vi "conti_move_v2.0.vi"(7 "enable":bool, 8 "error in (no error)":errorcluster, 9 "Position":T1, 11 "route":T2[](array[typedef])) -> (0 "error out":errorcluster, 1 "Position out":T1)   [LabVIEW 2019]
uses:
  move_cluster.ctl
  move/position cluster.ctl
  <vilib>/Platform/TimedLoop/XDataNode/timing_clust.ctl
  <vilib>/Platform/TimedLoop/XDataNode/nitl_modes.ctl
  <vilib>/Platform/TimedLoop/XDataNode/wakeup.ctl
  <vilib>/platform/TimedLoop/XDataNode/XDataNode.xnode
  <vilib>/Platform/TimedLoop/XDataNode/XDNodeRunTimeDep.lvlib
panel:
  out "Waveform Chart":cluster{"yaw":dbl, dbl}(graph)
  out "x-y":u32
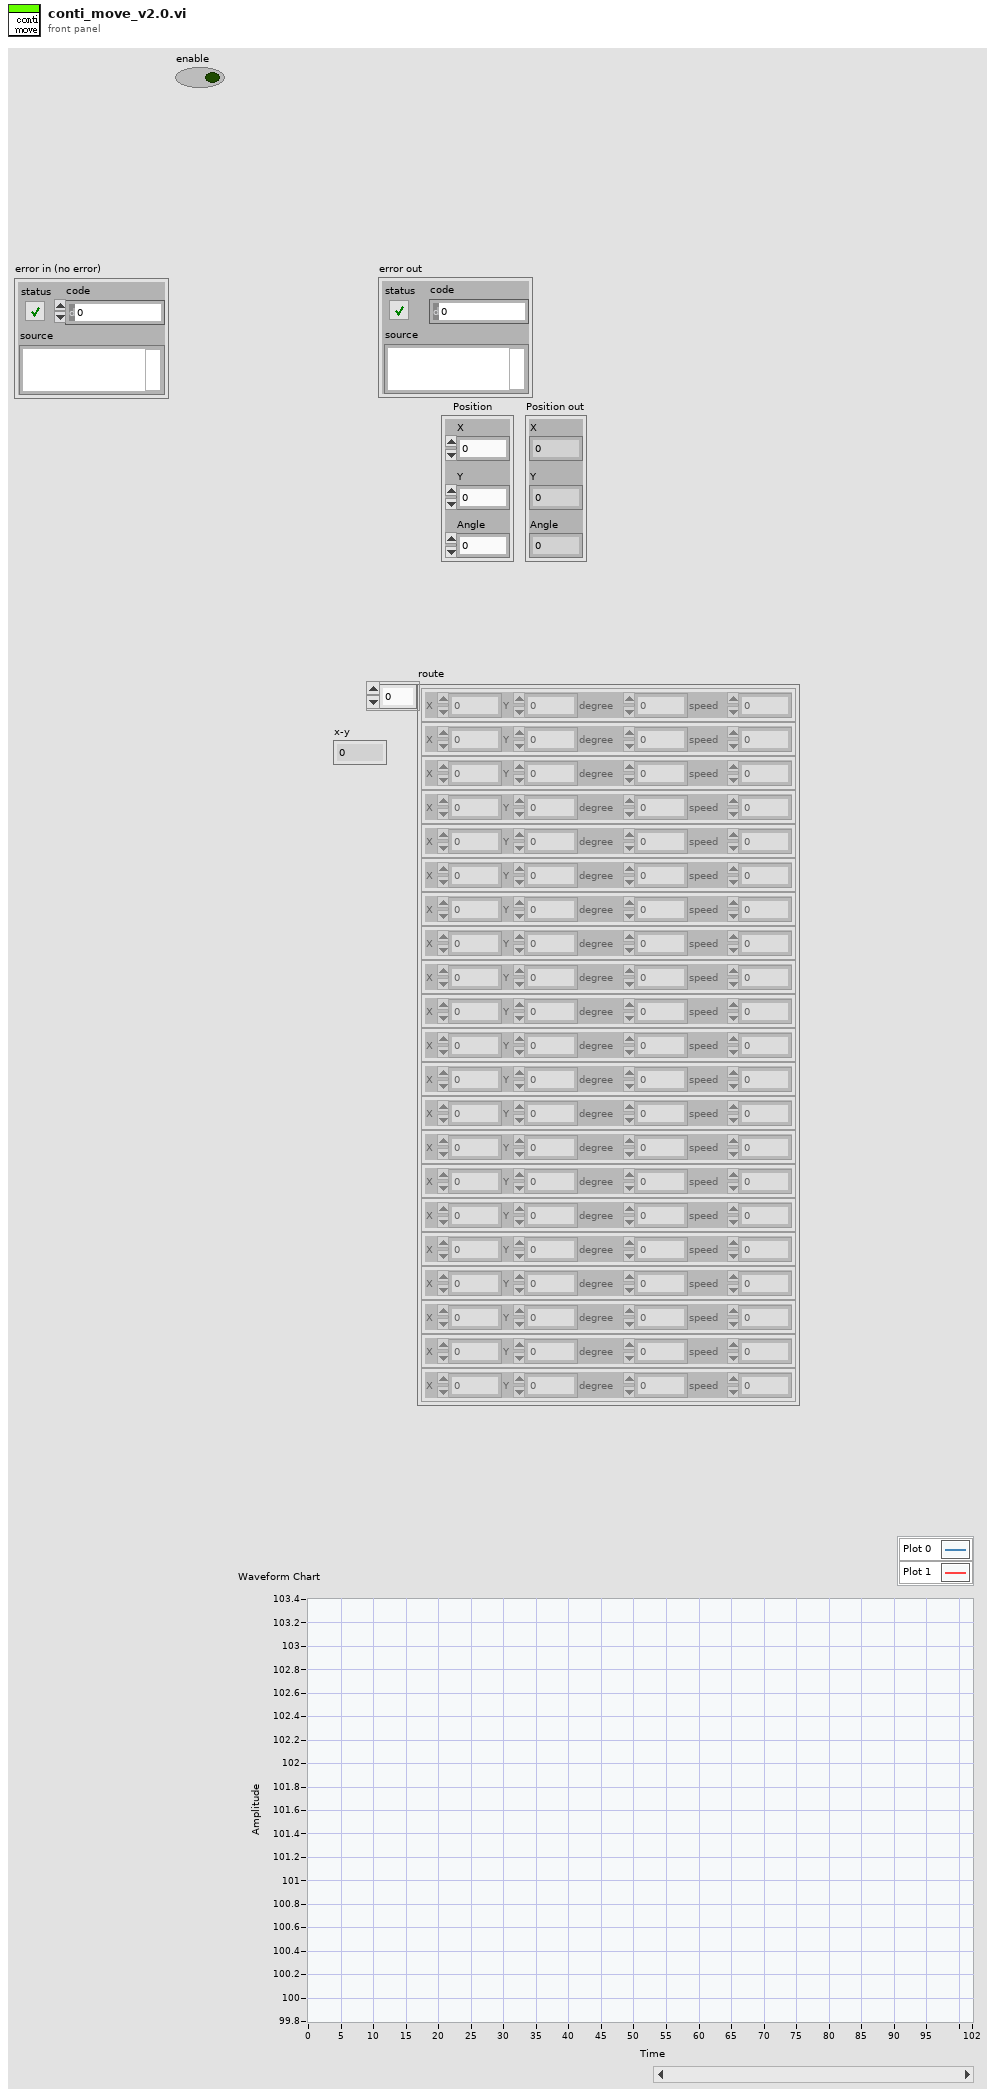
[diagram p1: front panel]
types:
  T1 = typedef "position cluster.ctl" = cluster{"X":dbl, "Y":dbl, "Angle":dbl}
  T2 = typedef "move_cluster.ctl" = cluster{"X":dbl, "Y":dbl, "degree":dbl, "speed":dbl}
  T3 = typedef "BNO055 gyro 3axis.ctl" = cluster{"yaw":dbl, "pitch":dbl, "roll":dbl}
  T4 = typedef "XDNodeRunTimeDep.lvlib/timing_clust.ctl" = cluster{"Expected End [f-1]":u64, "Actual End [f-1]":u64, "Finished Late? [f-1]":bool, "Expected End [i-1]":u64, "Actual End [i-1]":u64, "Finished Late? [i-1]":bool, "Expected Start [i]":u64, "Actual Start [i]":u64, "Expected Start [f]":u64, "Actual Start [f]":u64, "Source Name":string, "Structure Name":string, "Period":i64, "Deadline":i64, "Offset":i64, "Start":i64, "Priority":i32, "Timeout":i32, "Mode":T5, "Wakeup Reason":T6, "Error":errorcluster, "Source Type":string, "Secondary Source Type":string, "Global End Time":u64, "Global Start Time":u64, "Frame Duration":u64, "Iteration Duration":u64, "Assigned CPU":i32, "I/O Scan Engine Mode":u32}
  T5 = typedef "XDNodeRunTimeDep.lvlib/nitl_modes.ctl" = enum32{"No Change", "Process missed periods, maintain original phase", "Discard missed periods, maintain original phase", "Process missed periods, ignore original phase", "Discard missed periods, ignore original phase"}
  T6 = typedef "XDNodeRunTimeDep.lvlib/wakeup.ctl" = enum32{"Normal", "Aborted", "Asynchronous wakeup", "Timing source error", "Timed loop error", "Timeout"}
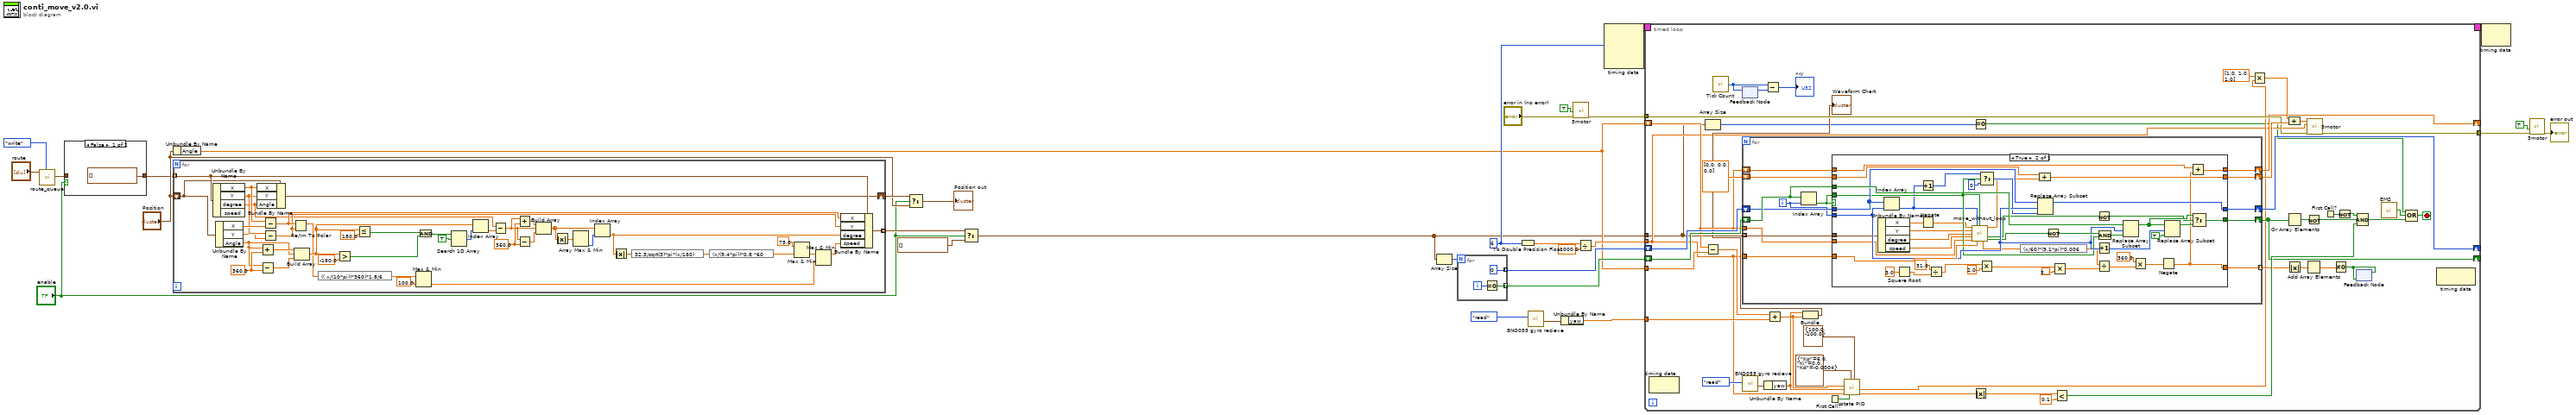
[diagram p0: block diagram]
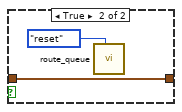
[diagram p2: hidden frame]
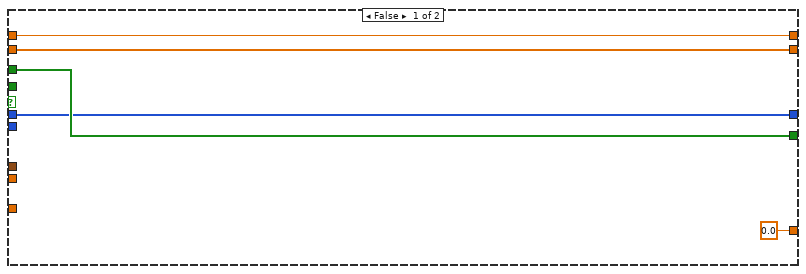
[diagram p3: hidden frame]
diagram:
  w27 = i64 6 ("Period")
  n1 = call "route_queue.vi"("set"=enum16{"reset", "write"}."write", "route"="route") -> ("read"=w2:T2[])  [unwired: 9 in]
  n2 = case shown="False" "enable" {
    tunnel: w2 -> [_ w33]
    tunnel: [T2[] [] ("read") w33] -> w3
    frame False {
    }
    frame True {
      n3 = call "route_queue.vi"("set"=enum16{"reset", "write"}."reset") -> ()  [unwired: 10 in, 1 out]
    }
  }
  n4 = Unbundle By Name("Position") -> ("Angle"=w12:dbl)
  n5 = for {
    tunnel: w3 -> [w75] mode=indexing
    tunnel: [w74] -> w9 mode=indexing
    shift-right: [w39] -> w10
    shift-left: "Position" -> [w73]
    w61 = 360.0
    w72 = 360.0
    n6 = Unbundle By Name(w75) -> ("X"=w53:dbl, "Y"=w51:dbl, "degree"=w38:dbl)  [unwired: 1 out]
    n7 = Unbundle By Name(w73) -> ("X"=w52:dbl, "Y"=w50:dbl, "Angle"=w54:dbl)
    n8 = Bundle By Name(cluster=w73, "X"=w53, "Y"=w51, "Angle"=w38) -> (w39:T1)
    n9 = Add(x=w54, y=w72) -> (x+y=w71:dbl)
    n10 = Subtract(x=w54, y=w72) -> (x-y=w70:dbl)
    n11 = Subtract(x=w53, y=w52) -> (x-y=w46:dbl)
    n12 = Subtract(x=w51, y=w50) -> (x-y=w45:dbl)
    n13 = Re/Im To Polar(2:w45, 3:w46) -> (1:w44:dbl)  [unwired: 1 out]
    n14 = Build Array(w71, w54, w70) -> (w62:dbl[])
    n15 = expression code="(( x/(10*pi))*360)*1.8/6"(w44) -> (w41:dbl)
    n16 = Greater?(x=w62, y=-180.0) -> (0:w66:bool[])
    n17 = Less Or Equal?(x=w62, y=180.0) -> (x <= y?=w67:bool[])
    n18 = Max & Min(x=w41, y=100.0) -> (min(x,y)=w36:dbl)  [unwired: 1 out]
    n19 = And(x=w67, y=w66) -> (x .and. y?=w65:bool[])
    n20 = Search 1D Array(1D array=w65, element=TRUE) -> (index of element=w63:i32)  [unwired: 1 in]
    n21 = Index Array(array=w62, index=w63) -> (element=w37:dbl)
    n22 = Subtract(x=w38, y=w37) -> (x-y=w59:dbl)
    n23 = Add(x=w59, y=w61) -> (x+y=w60:dbl)
    n24 = Subtract(x=w59, y=w61) -> (x-y=w58:dbl)
    n25 = Build Array(w60, w59, w58) -> (w55:dbl[])
    n26 = Absolute Value(x=w55) -> (abs(x)=w57:dbl[])
    n27 = Array Max & Min(array=w57) -> (min index (indices)=w56:i32)  [unwired: 3 out]
    n28 = Index Array(array=w55, index=w56) -> (element=w47:dbl)
    n29 = Absolute Value(x=w47) -> (abs(x)=w48:dbl)
    n30 = expression code="32.3/sqrt(3)*pi*(x/180)"(w48) -> (w49:dbl)
    n31 = expression code="(x/(9.4*pi))*0.8 *60"(w49) -> (w43:dbl)
    n32 = Max & Min(x=75.0, y=w43) -> (min(x,y)=w35:dbl)  [unwired: 1 out]
    n33 = Max & Min(x=w35, y=w36) -> (max(x,y)=w34:dbl)  [unwired: 1 out]
    n34 = Bundle By Name(cluster=w75, "X"=w46, "Y"=w45, "degree"=w47, "speed"=w34) -> (w74:T2)
  }
  n35 = Select(t=w10, s="enable", f="Position") -> (s? t:f=→"Position out":T1)
  n36 = Select(t=w9, s="enable", f=T2[] []) -> (s? t:f=w1:T2[])
  n37 = Array Size(array=w1) -> (size(s)=w23:i32)
  n38 = for {
    N: w23 -> [_]
    tunnel: [w76] -> w24 mode=indexing
    tunnel: [0 ("Boolean")] -> w22 mode=indexing
    i -> [w77]
    n39 = Equal To 0?(x=w77) -> (x = 0?=w76:bool)
  }
  n40 = To Double Precision Float(number=w27) -> (double precision float=w28:dbl)
  n41 = call "BNO055 gyro recieve.vi"("Enum"=enum16{"read", "write"}."read") -> ("read"=w14:T3)  [unwired: 10 in]
  n42 = Unbundle By Name(w14) -> ("yaw"=w13:dbl)
  n43 = call "3motor.vi"("error in (no error)"="error in (no error)", "Reset"=TRUE) -> ("error out"=w19:errorcluster)  [unwired: 8 in, 1 out]
  n44 = Divide(x=w28, y=1000.0) -> (x/y=w25:dbl)
  n45 = node-c288(w27) -> (w30:T4)  [unwired: 3 in]
  n46 = timed-loop {
    timing: w30 -> [_]
    timing-out: [_] -> w29
    tunnel: w25 -> [w82]
    shift-right: [w103] -> _
    shift-left: w24 -> [w125]
    shift-right: [w123] -> _
    shift-left: w22 -> [w124]
    shift-right: [w96] -> _
    shift-left: w12 -> [w111]
    tunnel: w1 -> [w81]
    tunnel: [w121] -> w21
    tunnel: w19 -> [w112]
    tunnel: w13 -> [w92]
    tunnel: w12 -> [w88]
    stop <- w117 stop-if-true
    n47 = node-c288() -> ()  [unwired: 1 in, 1 out]
    n48 = Array Size(array=w81) -> (size(s)=w80:i32)
    n49 = Subtract(x=w111, y=w88) -> (x-y=w89:dbl)
    n50 = call "Tick Count"() -> ("Tick Count(uSec)"=w106:u32)
    n51 = feedback-in #1(w106) -> ()
    n52 = feedback #1() -> (w105:u32)  [unwired: 1 in]
    n53 = for {
      tunnel: w82 -> [w139]
      shift-right: [w136] -> w103
      shift-left: w125 -> [w138]
      shift-right: [w132] -> w123
      shift-left: w124 -> [w137]
      shift-right: [w134] -> w120
      shift-left: dbl[] [0.0, 0.0, 0.0] -> [w133]
      shift-right: [w131] -> w96
      shift-left: w111 -> [w129]
      tunnel: w81 -> [w130] mode=indexing
      tunnel: [w128] -> w100 mode=indexing
      tunnel: w111 -> [w127]
      i -> [w135]
      n54 = Index Array(array=w138, index=w135) -> (element=w126:bool)
      n55 = case shown="True" w126 {
        tunnel: w139 -> [_ w190]
        tunnel: w138 -> [w144 w189]
        tunnel: w137 -> [w143 w188]
        tunnel: [w144 w186] -> w136
        tunnel: w135 -> [_ w181]
        tunnel: [w142 w178] -> w134
        tunnel: w133 -> [w142 w177]
        tunnel: w126 -> [_ w175]
        tunnel: [w143 w172] -> w132
        tunnel: [w141 w164] -> w131
        tunnel: w130 -> [_ w162]
        tunnel: w129 -> [w141 w149]
        tunnel: [0.0 w148] -> w128
        tunnel: w127 -> [_ w145]
        frame False {
        }
        frame True {
          n56 = Unbundle By Name(w162) -> ("X"=w147:dbl, "Y"=w160:dbl, "degree"=w159:dbl, "speed"=w161:dbl)
          n57 = Index Array(array=w188, index=w181) -> (element=w173:i32)
          n58 = Square Root(x=3.0) -> (sqrt(x)=w170:dbl)
          n59 = Increment(x=w173) -> (x+1=w174:i32)
          n60 = Negate(x=w147) -> (-x=w146:dbl)
          n61 = Divide(x=31.0, y=w170) -> (x/y=w168:dbl)
          n62 = call "move_without_loop.vi"("X"=w146, "i"=w173, "run"=w175, "Y"=w160, "deg"=w159, "speed"=w161, "offset"=w145, "dt"=w190) -> ("speed out"=w156:dbl[], "t2?"=w179:bool, "rotate speed"=w154:dbl, "complet"=w157:bool)  [unwired: 3 in, 1 out]
          n63 = Multiply(x=w168, y=2.0) -> (x*y=w165:dbl)
          n64 = Select(t=w174, s=w175, f=0) -> (s? t:f=w176:i32)
          n65 = expression code="(x/60)*(9.1*pi)*0.006"(w154) -> (w152:dbl)
          n66 = Replace Array Subset(array=w188, new element=w176, index=w181) -> (w172:i32[])
          n67 = Compound Arithmetic op=ADD(w177, w156) -> (w178:dbl[])
          n68 = Not(x=w157) -> (.not. x?=w187:bool)
          n69 = Multiply(x=w165, y=3.141592653589793) -> (x*y=w153:dbl)
          n70 = Not(x=w179) -> (.not. x?=w183:bool)
          n71 = Increment(x=w181) -> (x+1=w182:i32)
          n72 = Divide(x=w152, y=w153) -> (x/y=w163:dbl)
          n73 = Compound Arithmetic op=AND(w187, w175) -> (w158:bool)
          n74 = Replace Array Subset(array=w189, new element=w158, index=w181) -> (w185:bool[])
          n75 = Multiply(x=360.0, y=w163) -> (x*y=w151:dbl)
          n76 = Negate(x=w151) -> (-x=w148:dbl)
          n77 = Replace Array Subset(array=w185, new element=TRUE, index=w182) -> (w184:bool[])
          n78 = Add(x=w149, y=w148) -> (x+y=w164:dbl)
          n79 = Select(t=w185, s=w183, f=w184) -> (s? t:f=w186:bool[])
        }
      }
    }
    n80 = call "BNO055 gyro recieve.vi"("Enum"=enum16{"read", "write"}."read") -> ("read"=w91:T3)  [unwired: 10 in]
    n81 = Unbundle By Name(w91) -> ("yaw"=w85:dbl)
    n82 = Subtract(x=w106, y=w105) -> (x-y=→"x-y":u32)
    n83 = Add(x=w89, y=w92) -> (x+y=w84:dbl)
    n84 = Bundle("yaw"=w85, w84) -> (→"Waveform Chart":cluster{"yaw":dbl, dbl})  [unwired: 1 in]
    n85 = First Call?() -> (First Call?: T/F=w93:bool)
    n86 = call "rotate PID.vi"("output range"=cluster{"output high":dbl, "output low":dbl} {"output high"=100.0, "output low"=-100.0}, "s"=w93, "PID"=cluster{"Kp":dbl, "Ki":dbl, "Kd":dbl} {"Kp"=6.0, "Ki"=0.0, "Kd"=-0.0004}, "dt (s)"=w82, "Processer"=w85, "setpoint"=w84) -> ("e(t)"=w83:dbl, "out"=w87:dbl)  [unwired: 4 in]
    n87 = Equal To 0?(x=w80) -> (x = 0?=w79:bool)
    n88 = Absolute Value(x=w83) -> (abs(x)=w110:dbl)
    n89 = Less?(x=w110, y=0.1) -> (x < y?=w108:bool)
    n90 = Multiply(x=dbl[] [1.0, 1.0, 1.0], y=w87) -> (x*y=w118:dbl[])
    n91 = Or Array Elements(Boolean array=w103) -> (logical OR=w102:bool)
    n92 = Absolute Value(x=w100) -> (abs(x)=w99:dbl[])
    n93 = Compound Arithmetic op=ADD(w118, w120) -> (w107:dbl[])
    n94 = Add Array Elements(numeric array=w99) -> (sum=w98:dbl)
    n95 = Not(x=w102) -> (.not. x?=w101:bool)
    n96 = call "3motor.vi"("error in (no error)"=w112, "dt(s)"=w82, "Motor speed"=w107) -> ("error out"=w121:errorcluster)  [unwired: 7 in, 1 out]
    n97 = First Call?() -> (First Call?: T/F=w114:bool)
    n98 = Not Equal To 0?(x=w98) -> (x != 0?=w97:bool)
    n99 = Not(x=w114) -> (.not. x?=w113:bool)
    n100 = feedback-in #2(w97) -> ()
    n101 = feedback #2(w97) -> ()  [unwired: 1 in]
    n102 = Compound Arithmetic op=AND(w113, w101, w108) -> (w115:bool)
    n103 = call "EMS.vi"() -> ("A/DIO4 (Pin 19)"=w116:bool)
    n104 = Compound Arithmetic op=OR(w79, w116, w115) -> (w117:bool)
    n105 = node-c288() -> ()  [unwired: 1 in, 1 out]
  }
  n106 = node-c288(w29) -> ()  [unwired: 1 out]
  n107 = call "3motor.vi"("error in (no error)"=w21, "Reset"=TRUE) -> ("error out"=→"error out":errorcluster)  [unwired: 8 in, 1 out]
